vi "Check_Loop_Order.vi"(0 "Input Sequence":cluster{string, string[], dbl[], dbl}[](array[cluster])) -> (1 "Syntax Error":bool, 2 "Error Index":i32)   [LabVIEW 2011]
doc: "This VI checks to ensure that all loops and discrete API commands have \"end\" cases after their \"start\" cases."
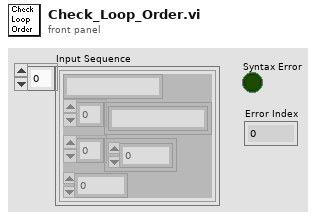
[diagram p1: front panel]
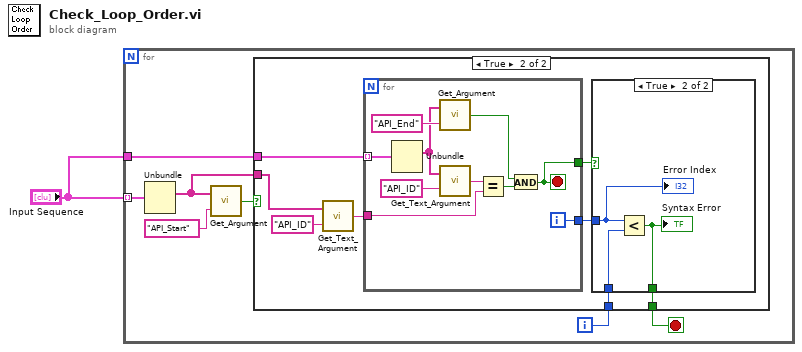
[diagram p0: block diagram]
diagram:
  n1 = for {
    tunnel: "Input Sequence" -> [w8] mode=indexing
    tunnel: "Input Sequence" -> [w4]
    i -> [w3]
    stop <- w2 stop-if-true
    n2 = Unbundle(w8) -> (w5:string[])  [unwired: 3 out]
    n3 = call "Get_Argument.vi"("Argument"="API_Start", "Argument List"=w5) -> ("Enabled"=w6:bool)
    n4 = case shown="True" w6 {
      tunnel: w5 -> [_ w16]
      tunnel: w4 -> [_ w14]
      tunnel: w3 -> [_ w10]
      tunnel: [_ w9] -> w2
      frame False {
      }
      frame True {
        n5 = call "Get_Text_Argument.vi"("Argument"="API_ID", "Argument List"=w16) -> ("Text"=w13:string)
        n6 = for {
          tunnel: w14 -> [w29] mode=indexing
          tunnel: w13 -> [w24]
          tunnel: [w21] -> w12
          tunnel: [w20] -> w11
          i -> [w20]
          stop <- w21 stop-if-true
          n7 = Unbundle(w29) -> (w26:string[])  [unwired: 3 out]
          n8 = call "Get_Argument.vi"("Argument"="API_End", "Argument List"=w26) -> ("Enabled"=w23:bool)
          n9 = call "Get_Text_Argument.vi"("Argument"="API_ID", "Argument List"=w26) -> ("Text"=w25:string)
          n10 = Equal?(x=w25, y=w24) -> (x = y?=w22:bool)
          n11 = And(x=w23, y=w22) -> (x .and. y?=w21:bool)
        }
        n12 = case shown="True" w12 {
          tunnel: w11 -> [_ w18]
          tunnel: w10 -> [_ w19]
          tunnel: [_ w17] -> w9
          frame False {
          }
          frame True {
            n13 = Less?(x=w18, y=w19) -> (x < y?=w17:bool)
            "Syntax Error" <- w17
            "Error Index" <- w18
          }
        }
      }
    }
  }
